vi "Drive Train.vi"   [LabVIEW 2018]
uses:
  <vilib>/Rock Robotics/WPI/ThirdParty/Phoenix-LabVIEW/Motor Controller/Controls/CTRE_Phoenix_MotorControl_NeutralMode.ctl
  <vilib>/Rock Robotics/SystemInterfaces/AI/FPGA_AIChannel.ctl
  <vilib>/Rock Robotics/WPI/Counter/WPI_CounterDigitalInputToDigitalSource.vi
  <vilib>/Rock Robotics/SystemInterfaces/DIO/FPGA_DIOChannel.ctl
  Times/Times Global.vi
  Drive Train Global.vi
  <vilib>/Rock Robotics/WPI/ThirdParty/Sensors/navX/_TypeDefs/FRIC_navX_DeviceNumbersTypeDef.ctl
types:
  T1 = typedef "FPGA_AIChannel.ctl" = enum8{"AI 0", "AI 1", "AI 2", "AI 3", "AI MXP 0", "AI MXP 1", "AI MXP 2", "AI MXP 3", "Invalid"}
  T2 = typedef "FPGA_DIOChannel.ctl" = enum8{"DIO 0", "DIO 1", "DIO 2", "DIO 3", "DIO 4", "DIO 5", "DIO 6", "DIO 7", "DIO 8", "DIO 9", "DIO MXP 0", "DIO MXP 1", "DIO MXP 2", "DIO MXP 3", "DIO MXP 4", "DIO MXP 5", "DIO MXP 6", "DIO MXP 7", "DIO MXP 8", "DIO MXP 9", "DIO MXP 10", "DIO MXP 11", "DIO MXP 12", "DIO MXP 13", "DIO MXP 14", "DIO MXP 15", "SPI Port CS1", "SPI Port CS2", "SPI Port CS3", "SPI Port MISO", "SPI Port MOSI", "Invalid"}
  T3 = typedef "CTRE_Phoenix_MotorControl_NeutralMode.ctl" = enum8{"EEPROMSetting", "Override to Coast", "Override to Brake"}
  T4 = typedef "WPI_MotorControlDeviceRef.ctl" = cluster{"DeviceStatus":errorcluster, "Type":T5, "PWM":cluster{"PWM Channel":T6, "DeadBand":T7}, "CAN":cluster{"Device Number":u8, "SetOutput VI Ref":variant, "GetOutput VI Ref":variant, "Enable VI Ref":variant, "Disable VI Ref":variant, "Data":variant}, "Invert":bool, "DIO PWM":cluster{"PWM \"Enable\" Channel":T6, "DIOChannel":T2, "PWM Rate":dbl}}
  T5 = typedef "WPI_MotorControlType.ctl" = enum16{"PWM", "CAN", "DIO PWM"}
  T6 = typedef "FPGA_DIOPWMChannel.ctl" = enum8{"PWM 0", "PWM 1", "PWM 2", "PWM 3", "PWM 4", "PWM 5", "PWM 6", "PWM 7", "PWM 8", "PWM 9", "PWM MXP 0", "PWM MXP 1", "PWM MXP 2", "PWM MXP 3", "PWM MXP 4", "PWM MXP 5", "PWM MXP 6", "PWM MXP 7", "PWM MXP 8", "PWM MXP 9", "Invalid"}
  T7 = typedef "WPI_PWMDeadband.ctl" = cluster{"Name":string, "maxPositivePwm":i32, "minPositivePwm":i32, "centerPwm":i32, "maxNegativePwm":i32, "minNegativePwm":i32, "angularRange":u16}
  T8 = typedef "WPI_DigitalInputDevRef.ctl" = cluster{"DevStatus":errorcluster, "DIO Channel":T2}
  T9 = typedef "WPI_PotentiometerDevRef.ctl" = cluster{"DevStatus":errorcluster, "Analog Channel":T1, "Invert Output":bool}
  T10 = typedef "FPGA_CounterEncoderSourceConvertionLVSourceType.ctl" = cluster{"DevStatus":errorcluster, "AnalogTriggerMode?":bool, "DigitalMode":cluster{"DIO Channel":T11}, "AnalogTriggerMode":cluster{"AnalogTriggerIndex":T12, "OutputType":T13}}
  T11 = typedef "FPGA_DIODigitalSourceChannel.ctl" = enum8{"DIO 0", "DIO 1", "DIO 2", "DIO 3", "DIO 4", "DIO 5", "DIO 6", "DIO 7", "DIO 8", "DIO 9", "DIO MXP 0", "DIO MXP 1", "DIO MXP 2", "DIO MXP 3", "DIO MXP 4", "DIO MXP 5", "DIO MXP 6", "DIO MXP 7", "DIO MXP 8", "DIO MXP 9", "DIO MXP 10", "DIO MXP 11", "DIO MXP 12", "DIO MXP 13", "DIO MXP 14", "DIO MXP 15", "SPI Port CS1", "SPI Port CS2", "SPI Port CS3", "SPI Port MISO", "SPI Port MOSI", "Disabled"}
  T12 = typedef "FPGA_AnalogTriggerIndex.ctl" = enum8{"Trig 0", "Trig 1", "Trig 2", "Trig 3", "Trig 4", "Trig 5", "Trig 6", "Trig 7", "Invalid"}
  T13 = typedef "FPGA_AnalogTriggerOutType.ctl" = enum16{"InWindow", "TriggerState", "Rising", "Falling"}
  T14 = typedef "WPI_EncoderDevRef.ctl" = cluster{"DevStatus":errorcluster, "EncoderIndex":T15, "CounterIndex":T16, "DistancePerCount":dbl, "Decoding Type":T17}
  T15 = typedef "FPGA_EncoderIdx.ctl" = enum8{"Enc 0", "Enc 1", "Enc 2", "Enc 3", "Enc 4", "Enc 5", "Enc 6", "Enc 7", "Invalid"}
  T16 = typedef "FPGA_CounterCtrSystemIndex.ctl" = enum8{"Ctr 0", "Ctr 1", "Ctr 2", "Ctr 3", "Ctr 4", "Ctr 5", "Ctr 6", "Ctr 7", "Invalid"}
  T17 = typedef "WPI_EncoderType.ctl" = enum16{"1x", "2x", "4x"}
  T18 = typedef "FRIC_navX_DeviceNumbersTypeDef.ctl" = enum16{"Dev0", "Dev1", "Dev2", "Dev3"}
  T19 = typedef "Control 2.ctl" = dbl
  T20 = cluster{"Rollover":dbl, "Yaw":dbl, "Cont Yaw":dbl}
  T21 = cluster{"FrontLeft":dbl, "FrontRight":dbl, "BackLeft":dbl, "BackRight":dbl}
  T22 = enum16{"Back Left", "Back Right", "Front Left", "Front Right"}
  T23 = enum16{"Autonomous Mode", "Field Oriented", "Robot Oriented", "Tank Mode"}
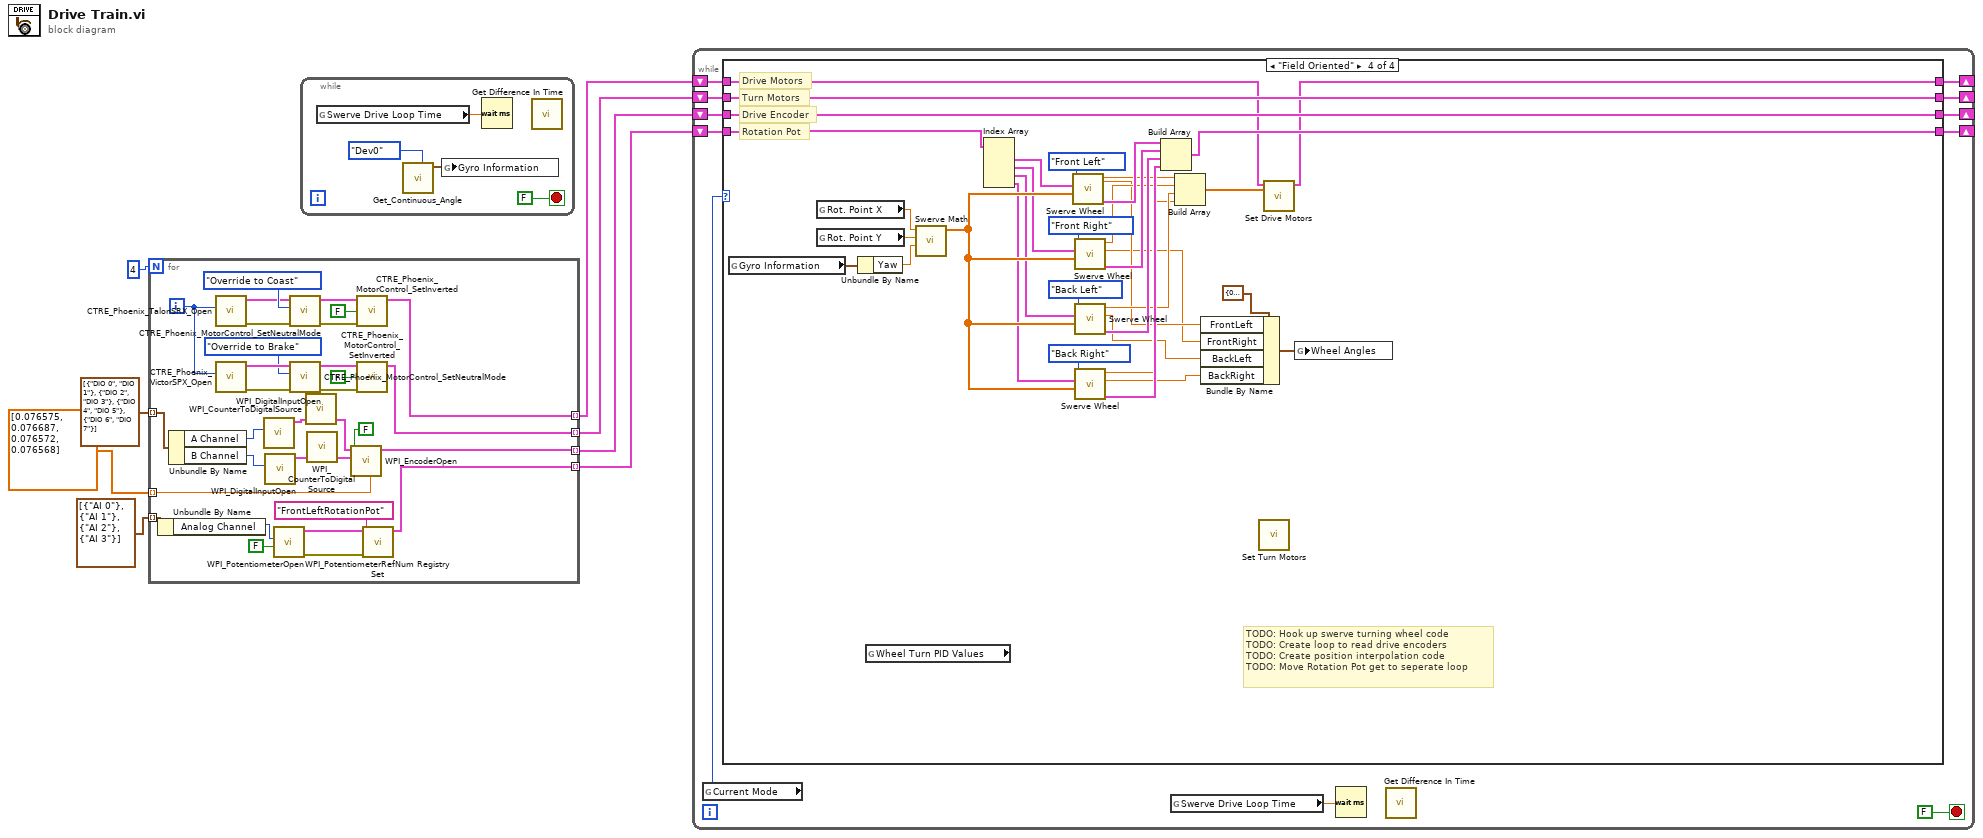
[diagram p0: block diagram]
diagram:
  n1 = for {
    N: 4 -> [_]
    tunnel: cluster{"A Channel":T2, "B Channel":T2}[] [{"A Channel"=enum."DIO 0", "B Channel"=enum."DIO 1"}, {"A Channel"=enum."DIO 2", "B Channel"=enum."DIO 3"}, {"A Channel"=enum."DIO 4", "B Channel"=enum."DIO 5"}, {"A Channel"=enum."DIO 6", "B Channel"=enum."DIO 7"}] -> [w18] mode=indexing
    tunnel: cluster{"Analog Channel":T1}[] [{"Analog Channel"=enum."AI 0"}, {"Analog Channel"=enum."AI 1"}, {"Analog Channel"=enum."AI 2"}, {"Analog Channel"=enum."AI 3"}] -> [w15] mode=indexing
    tunnel: dbl[] [0.076575, 0.076687, 0.076572, 0.076568] -> [w13] mode=indexing
    tunnel: [w12] -> w4 mode=indexing
    tunnel: [w11] -> w3 mode=indexing
    tunnel: [w10] -> w2 mode=indexing
    tunnel: [w9] -> w1 mode=indexing
    i -> [w19]
    n2 = Unbundle By Name(w15) -> ("Analog Channel"=w14:T1)
    n3 = Unbundle By Name(w18) -> ("A Channel"=w17:T2, "B Channel"=w16:T2)
    n4 = call <vilib>:"CTRE_Phoenix_TalonSRX_Open.vi"("Device Number"=w19) -> ("error out"=w20:errorcluster, "CAN Talon SRX Ref"=w21:T4)  [unwired: 9 in]
    n5 = call <vilib>:"CTRE_Phoenix_VictorSPX_Open.vi"("Device Number"=w19) -> ("error out"=w31:errorcluster, "CAN Talon SRX Ref"=w30:T4)  [unwired: 9 in]
    n6 = call <vilib>:"WPI_DigitalInputOpen.vi"("DIO Channel"=w17) -> ("DigitalInputDevRef"=w38:T8)  [unwired: 1 in, 9 out]
    n7 = call <vilib>:"WPI_DigitalInputOpen.vi"("DIO Channel"=w16) -> ("DigitalInputDevRef"=w37:T8)  [unwired: 1 in, 9 out]
    n8 = call <vilib>:"WPI_PotentiometerOpen.vi"("Invert Output"=FALSE, "Analog Channel"=w14) -> ("error out"=w33:errorcluster, "PotDevRef"=w34:T9)  [unwired: 8 in]
    n9 = call <vilib>:"CTRE_Phoenix_MotorControl_SetNeutralMode.vi"("error in (no error)"=w20, "Motor Control Neutral Mode"=CTRE_Phoenix_MotorControl_NeutralMode."Override to Coast", "PhoenixMotorControlDevRef"=w21) -> ("error out"=w23:errorcluster, "PhoenixMotorControlDevRef"=w24:T4)  [unwired: 7 in]
    n10 = call <vilib>:"CTRE_Phoenix_MotorControl_SetNeutralMode.vi"("error in (no error)"=w31, "Motor Control Neutral Mode"=CTRE_Phoenix_MotorControl_NeutralMode."Override to Brake", "PhoenixMotorControlDevRef"=w30) -> ("error out"=w28:errorcluster, "PhoenixMotorControlDevRef"=w27:T4)  [unwired: 7 in]
    n11 = call-poly <vilib>:"WPI_CounterToDigitalSource.vi"("DigitalInputDevRef"=w38) -> ("Digital Source"=w39:T10)  [unwired: 6 out]
    n12 = call-poly <vilib>:"WPI_CounterToDigitalSource.vi"("DigitalInputDevRef"=w37) -> ("Digital Source"=w36:T10)  [unwired: 6 out]
    n13 = call <vilib>:"WPI_EncoderOpen.vi"("DistancePerCount"=w13, "Invert Direction (False)"=FALSE, "BSource"=w36, "ASource"=w39) -> ("EncoderDevRef"=w10:T14)  [unwired: 4 in, 3 out]
    n14 = call <vilib>:"CTRE_Phoenix_MotorControl_SetInverted.vi"("error in (no error)"=w23, "Invert?"=FALSE, "PhoenixMotorControlDevRef"=w24) -> ("PhoenixMotorControlDevRef"=w12:T4)  [unwired: 7 in, 1 out]
    n15 = call <vilib>:"CTRE_Phoenix_MotorControl_SetInverted.vi"("error in (no error)"=w28, "Invert?"=FALSE, "PhoenixMotorControlDevRef"=w27) -> ("PhoenixMotorControlDevRef"=w11:T4)  [unwired: 7 in, 1 out]
    n16 = call <vilib>:"WPI_PotentiometerRefNum Registry Set.vi"("error in (no error)"=w33, "refnum name"="FrontLeftRotationPot", "PotDevRef"=w34) -> ("PotDevRef"=w9:T9)  [unwired: 7 in, 1 out]
  }
  n17 = while {
    stop <- FALSE stop-if-true
    n18 = global read "Times Global.vi" "Swerve Drive Loop Time"() -> (w41:T19)
    n19 = call <vilib>:"Get_Continuous_Angle.vi"("Device Number"=FRIC_navX_DeviceNumbersTypeDef."Dev0") -> ("Continuous Angle"=w42:T20)  [unwired: 10 in]
    n20 = global write "Drive Train Global.vi" "Gyro Information"(w42) -> ()
    n21 = Wait (ms)(milliseconds to wait=w41) -> ()  [unwired: 1 out]
    n22 = call "Get Difference In Time.vi"() -> ()  [unwired: 10 in, 2 out]
  }
  n23 = while {
    shift-right: [w48] -> _
    shift-left: w4 -> [w52]
    shift-right: [w47] -> _
    shift-left: w3 -> [w51]
    shift-right: [w46] -> _
    shift-left: w2 -> [w50]
    shift-right: [w45] -> _
    shift-left: w1 -> [w49]
    stop <- FALSE stop-if-true
    n24 = global read "Drive Train Global.vi" "Current Mode"() -> (w53:T23)
    n25 = case shown="\"Field Oriented\"" w53 {
      tunnel: w52 -> [w59 w63 w67 w75]
      tunnel: w51 -> [w58 w62 w66 w97]
      tunnel: w50 -> [w57 w61 w65 w96]
      tunnel: w49 -> [w56 w60 w64 w86]
      tunnel: [w59 w63 w67 w74] -> w48
      tunnel: [w58 w62 w66 w97] -> w47
      tunnel: [w57 w61 w65 w96] -> w46
      tunnel: [w56 w60 w64 w85] -> w45
      frame "Autonomous Mode", Default {
        # "Rotation Pot"
        # "Drive Encoder"
        # "Turn Motors"
        # "Drive Motors"
      }
      frame "Robot Oriented" {
        # "Rotation Pot"
        # "Drive Encoder"
        # "Turn Motors"
        # "Drive Motors"
      }
      frame "Tank Mode" {
        # "Rotation Pot"
        # "Drive Encoder"
        # "Turn Motors"
        # "Drive Motors"
      }
      frame "Field Oriented" {
        # "TODO: Hook up swerve turning wheel code\nTODO: Create loop to read drive encoders\nTODO: Create position interpolation code\nTODO: Move Rotation Pot get to seperate loop"
        # "Rotation Pot"
        # "Drive Encoder"
        # "Turn Motors"
        # "Drive Motors"
        n26 = global read "Drive Train Global.vi" "Gyro Information"() -> (w94:T20)
        n27 = global read "Drive Train Global.vi" "Rot. Point X"() -> (w93:dbl)
        n28 = global read "Drive Train Global.vi" "Rot. Point Y"() -> (w92:dbl)
        n29 = Unbundle By Name(w94) -> ("Yaw"=w91:dbl)
        n30 = global read "Drive Train Global.vi" "Wheel Turn PID Values"() -> ()  [unwired: 1 out]
        n31 = call "Swerve Math.vi"("Yaw"=w91, "Rot. Point Y"=w92, "Rot. Point X"=w93) -> ("Swerve Math Ouput"=w95:dbl[])  [unwired: 8 in]
        n32 = Index Array(array=w86) -> (element #1=w90:T9, element #2=w89:T9, element #3=w88:T9, element #4=w87:T9)  [unwired: 4 in]
        n33 = call "Swerve Wheel.vi"("Inputs"=w95, "Pot Ref In"=w90, "Wheel"=T22."Front Left") -> ("Pot Ref Out"=w81:T9, "Wheel Angle"=w72:dbl, "Speed"=w80:dbl)  [unwired: 5 in, 1 out]
        n34 = call "Swerve Wheel.vi"("Inputs"=w95, "Pot Ref In"=w89, "Wheel"=T22."Front Right") -> ("Pot Ref Out"=w82:T9, "Wheel Angle"=w71:dbl, "Speed"=w79:dbl)  [unwired: 5 in, 1 out]
        n35 = call "Swerve Wheel.vi"("Inputs"=w95, "Pot Ref In"=w88, "Wheel"=T22."Back Left") -> ("Pot Ref Out"=w83:T9, "Wheel Angle"=w70:dbl, "Speed"=w78:dbl)  [unwired: 5 in, 1 out]
        n36 = call "Swerve Wheel.vi"("Inputs"=w95, "Pot Ref In"=w87, "Wheel"=T22."Back Right") -> ("Pot Ref Out"=w84:T9, "Wheel Angle"=w69:dbl, "Speed"=w77:dbl)  [unwired: 5 in, 1 out]
        n37 = Build Array(w81, w82, w83, w84) -> (w85:T9[])
        n38 = Build Array(w80, w79, w78, w77) -> (w76:dbl[])
        n39 = Bundle By Name(cluster=T21 {"FrontLeft"=0.0, "FrontRight"=0.0, "BackLeft"=0.0, "BackRight"=0.0} ("Wheel Angles"), "FrontLeft"=w72, "FrontRight"=w71, "BackLeft"=w70, "BackRight"=w69) -> (w68:T21)
        n40 = call "Set Turn Motors.vi"() -> ()  [unwired: 12 in]
        n41 = call "Set Drive Motors.vi"("appended array"=w76, "Motors In"=w75) -> ("Motors Out"=w74:T4[])  [unwired: 9 in]
        n42 = global write "Drive Train Global.vi" "Wheel Angles"(w68) -> ()
      }
    }
    n43 = global read "Times Global.vi" "Swerve Drive Loop Time"() -> (w54:T19)
    n44 = Wait (ms)(milliseconds to wait=w54) -> ()  [unwired: 1 out]
    n45 = call "Get Difference In Time.vi"() -> ()  [unwired: 10 in, 2 out]
  }
